vi "EditorMousePositionOverArray.vi"(8 "Coords":T3, 9 "Position":T2, 10 "Bounds":T1, 11 "Size(s)":i32[](array[numeric])) -> (3 "Indexes":cluster{"row":i32, "col":i32})   [LabVIEW 2020]
uses:
  <vilib>/Utility/miscctls.llb/LVPoint32TypeDef.ctl
  <vilib>/Utility/miscctls.llb/LVPositionTypeDef.ctl
  <vilib>/Utility/miscctls.llb/LVBoundsTypeDef.ctl
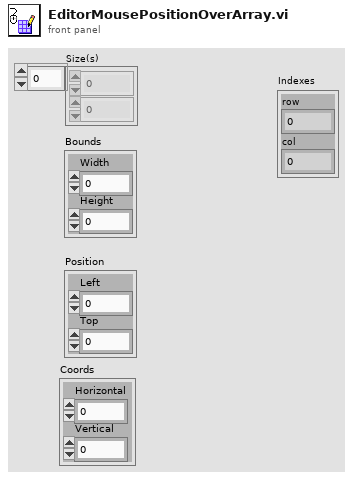
[diagram p1: front panel]
types:
  T1 = typedef "LVBoundsTypeDef.ctl" = cluster{"Width":u32, "Height":u32}
  T2 = typedef "LVPositionTypeDef.ctl" = cluster{"Left":i32, "Top":i32}
  T3 = typedef "LVPoint32TypeDef.ctl" = cluster{"Horizontal":i32, "Vertical":i32}
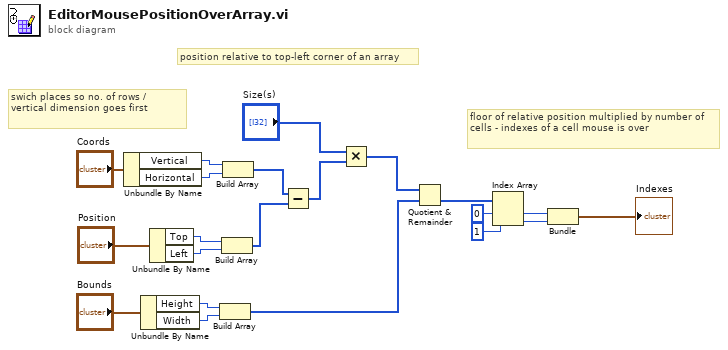
[diagram p0: block diagram]
diagram:
  # "floor of relative position multiplied by number of cells - indexes of a cell mouse is over"
  # "swich places so no. of rows / vertical dimension goes first"
  # "position relative to top-left corner of an array"
  n1 = Unbundle By Name("Coords") -> ("Vertical"=w18:i32, "Horizontal"=w17:i32)
  n2 = Unbundle By Name("Bounds") -> ("Height"=w14:u32, "Width"=w13:u32)
  n3 = Unbundle By Name("Position") -> ("Top"=w16:i32, "Left"=w15:i32)
  n4 = Build Array(w14, w13) -> (w7:u32[])
  n5 = Build Array(w16, w15) -> (w11:i32[])
  n6 = Build Array(w18, w17) -> (w12:i32[])
  n7 = Subtract(x=w12, y=w11) -> (x-y=w9:i32[])
  n8 = Multiply(x="Size(s)", y=w9) -> (x*y=w8:i32[])
  n9 = Quotient & Remainder(x=w8, y=w7) -> (floor(x/y)=w6:u32[])  [unwired: 1 out]
  n10 = Index Array(array=w6, index #1=0 ("index"), index #2=1 ("index")) -> (element #1=w2:u32, element #2=w3:u32)
  n11 = Bundle(w2, w3) -> (→"Indexes":cluster{u32, u32})  [unwired: 1 in]
